vi "Module.LaunchVI from Ref.vi"(0 "Parent Q":refnum<queue>, 1 "Ping Check":bool, 3 "Index":i32, 5 "VI Ref In":refnum<vi>, 9 "Q Name":string, 11 "error in":errorcluster, 12 "Working Dirs":T1, 13 "Simulate":bool, 14 "Error if Already Running":bool) -> (4 "VI Ref Out":refnum<vi>, 6 "Already Exists":bool, 15 "error out":errorcluster)   [LabVIEW 2024, in "EQMF.lvlib" / "Module Utils.lvlib"]
uses:
  Module Utils.lvlib
  Queues/Q.Element.ctl
  Module.Working Dirs.ctl
  Module Config.ctl
  Queues/Queue Utils.lvlib
panel:
  in  "Show Menu Bar(F)":bool
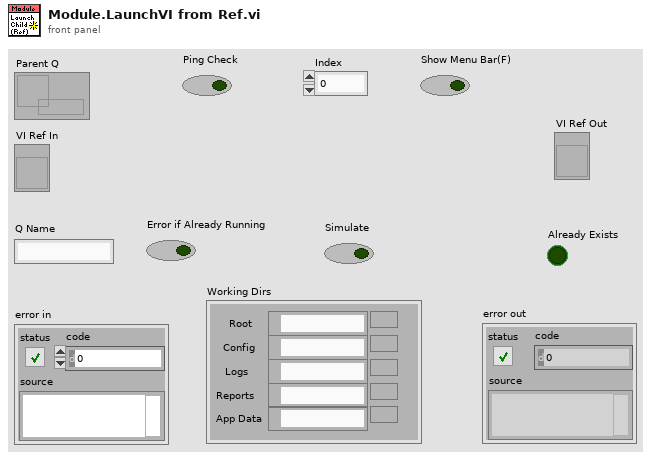
[diagram p1: front panel]
types:
  T1 = typedef "EQMF.lvlib/Module Utils.lvlib/Module.Working Dirs.ctl" = cluster{"Root":path, "Config":path, "Logs":path, "Reports":path, "App Data":path}
  T2 = typedef "EQMF.lvlib/Queue Utils.lvlib/Q.Element.ctl" = cluster{"Cmd":string, "Sub":string, "Data1":variant, "Data2":variant}
  T3 = typedef "EQMF.lvlib/Module Utils.lvlib/Module Config.ctl" = cluster{"Name":string, "Parent Q":refnum<queue>, "Is Child?":bool, "Index":i32, "Dirs":T1, "Simulate":bool, "SimCtrl":refnum<vi>}
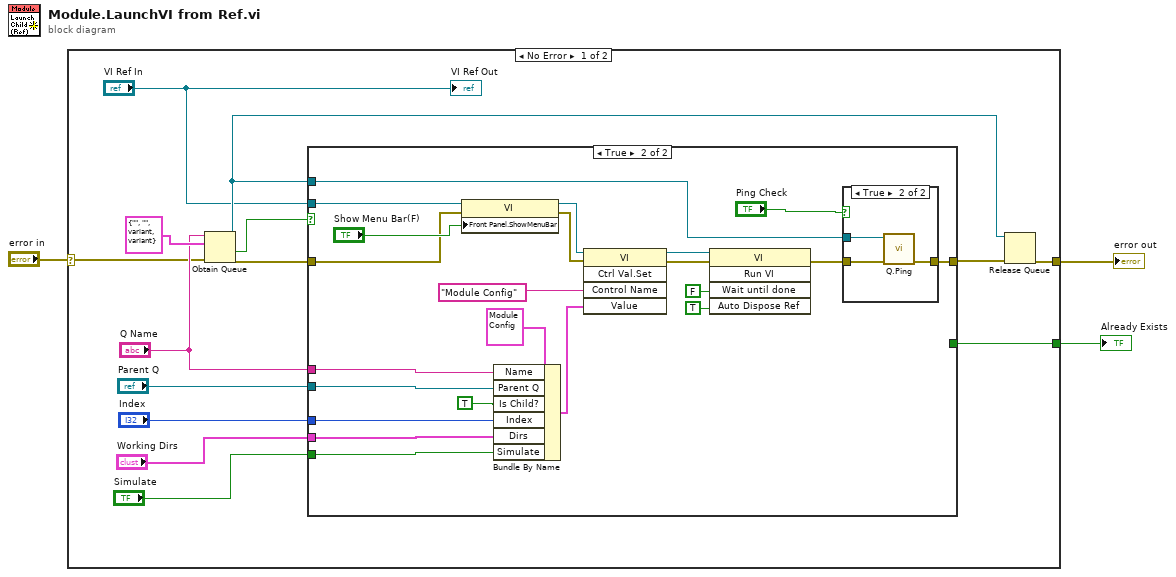
[diagram p0: block diagram]
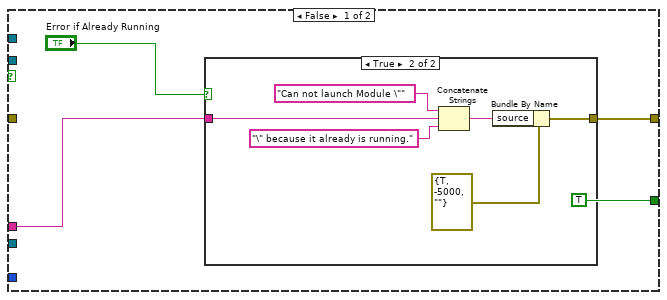
[diagram p2: hidden frame]
diagram:
  n1 = case shown="No Error" "error in" {
    selector: "error in" -> [w11 w54]
    tunnel: [w10 w54] -> w3
    tunnel: [w6 _] -> w1
    frame No Error {
      n2 = Obtain Queue(name (unnamed)="Q Name", element data type=T2 {"Cmd"="", "Sub"="", "Data1"=variant, "Data2"=variant} ("MainQ.Element"), error in (no error)=w11) -> (queue out=w7:refnum<queue>, created new?=w12:bool, error out=w8:errorcluster)  [unwired: 2 in]
      n3 = case shown="True" w12 {
        tunnel: w8 -> [_ w29]
        tunnel: "Q Name" -> [w21 w42]
        tunnel: "Parent Q" -> [_ w41]
        tunnel: "Index" -> [_ w39]
        tunnel: "Working Dirs" -> [_ w38]
        tunnel: [w20 w37] -> w9
        tunnel: w7 -> [_ w36]
        tunnel: [TRUE _] -> w6
        tunnel: "Simulate" -> [_ w33]
        tunnel: "VI Ref In" -> [_ w32]
        frame False {
          n4 = case shown="True" "Error if Already Running" {
            tunnel: w21 -> [_ w25]
            tunnel: [_ w24] -> w20
            frame False {
            }
            frame True {
              n5 = Concatenate Strings("Can not launch Module \"", w25, "\" because it already is running.") -> (w22:string)
              n6 = Bundle By Name(cluster=errorcluster {"status"=TRUE, "code"=-5000, "source"=""} ("error constant"), "source"=w22) -> (w24:errorcluster)
            }
          }
        }
        frame True {
          n7 = property class="VI"(reference=w32, error in=w29, "Front Panel.ShowMenuBar"="Show Menu Bar(F)") -> (reference out=w31:refnum<vi>, error out=w28:errorcluster)
          n8 = Bundle By Name(cluster=T3 {"Name"="", "Parent Q"=refnum, "Is Child?"=FALSE, "Index"=0, "Dirs"={"Root"=path "", "Config"=path "", "Logs"=path "", "Reports"=path "", "App Data"=path ""}, "Simulate"=FALSE, "SimCtrl"=refnum}, "Name"=w42, "Parent Q"=w41, "Is Child?"=TRUE ("Child"), "Index"=w39, "Dirs"=w38, "Simulate"=w33) -> (w43:T3)
          n9 = invoke class="VI" method="Ctrl Val.Set"(reference=w31, error in=w28, "Control Name"="Module Config", "Value"=w43) -> (reference out=w48:refnum<vi>, error out=w49:errorcluster)  [unwired: 1 in, 3 out]
          n10 = invoke class="VI" method="Run VI"(reference=w48, error in=w49, "Wait until done"=FALSE ("Wait Until Done"), "Auto Dispose Ref"=TRUE ("Auto Dispose Reference")) -> (error out=w35:errorcluster)  [unwired: 1 in, 4 out]
          n11 = case shown="True" "Ping Check" {
            tunnel: [w50 w53] -> w37
            tunnel: w36 -> [_ w52]
            tunnel: w35 -> [w50 w51]
            frame False {
            }
            frame True {
              n12 = call "Q.Ping.vi"("Error In"=w51, "Target Q In"=w52) -> ("Error Out"=w53:errorcluster)  [unwired: 6 in, 3 out]
            }
          }
        }
      }
      n13 = Release Queue(queue=w7, error in (no error)=w9) -> (error out=w10:errorcluster)  [unwired: 1 in, 2 out]
      "VI Ref Out" <- "VI Ref In"
    }
    frame Error {
    }
  }
  "error out" <- w3
  "Already Exists" <- w1
